vi "v5.vi"() -> ()   [LabVIEW 2022 SP3]
uses:
  <vilib>/DAQmx/read.llb/DAQmx Read (Analog 1D DBL NChan 1Samp).vi
  <vilib>/DAQmx/write.llb/DAQmx Write (Digital Bool 1Line 1Point).vi
  <vilib>/DAQmx/create/channels.llb/DAQmx Create Channel (AI-Voltage-Basic).vi
  <vilib>/DAQmx/create/channels.llb/DAQmx Create Channel (DO-Digital Output).vi
  <vilib>/DAQmx/miscellaneous.llb/DAQmx Fill In Error Info.vi
panel:
  out "Gas detected":bool
  out "flame detected":bool
  in  "lines":tag
  in  "VISA resource name 5":refnum<visa-resource-name>
  out "Fire detected (from camera)":bool
  out "number":i32
  out "data out":string
  in  "Play":bool
  out "Video":picture
  out "error out":errorcluster
  in  "Gas Sensor threshold":dbl
  in  "Temperature Threshold":dbl
  in  "IR sensor threshhold":dbl
  out "temperature voltage output":dbl
  out "MQ2 gas sensor":dbl(knob) scale=0.0..4.0
  out "IR sensor":dbl(knob) scale=2.0..4.0
  out "Temperature":dbl(knob) scale=10.0..60.0
  out "Gas sensor voltage output":dbl
  out "IR sensor voltage output":dbl
  out "Temperatue":dbl
  in  "VISA resource name 4":refnum<visa-resource-name>
  in  "VISA resource name 3":refnum<visa-resource-name>
  in  "VISA resource name":refnum<visa-resource-name>
  in  "VISA resource name 2":refnum<visa-resource-name>
  in  "stop":bool
  in  "physical channels":tag
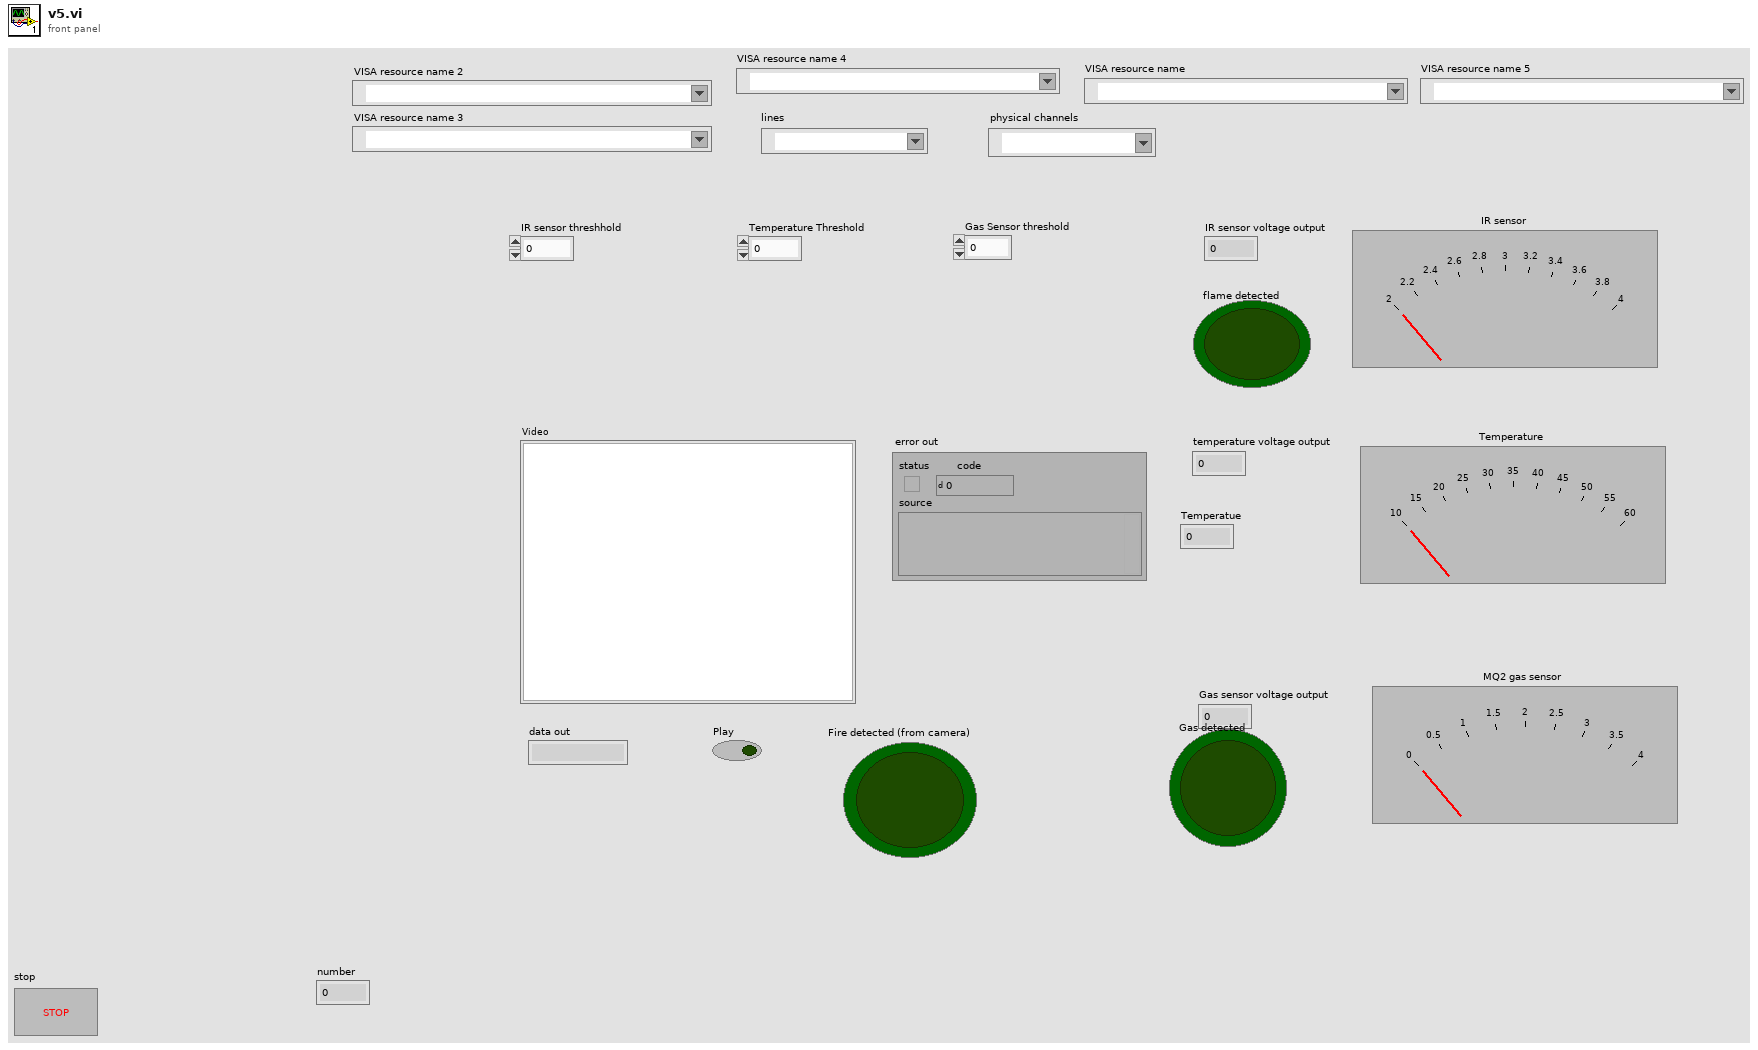
[diagram p1: front panel]
types:
  T1 = enum16{"open", "replace", "create", "open or create", "replace or create", "replace or create with confirmation"}
  T2 = typedef "imagedata.ctl" = cluster{"image type":i32, "image depth":i32, "image":u8[], "mask":u8[], "colors":u32[], "Rectangle":cluster{"left":i16, "top":i16, "right":i16, "bottom":i16}}
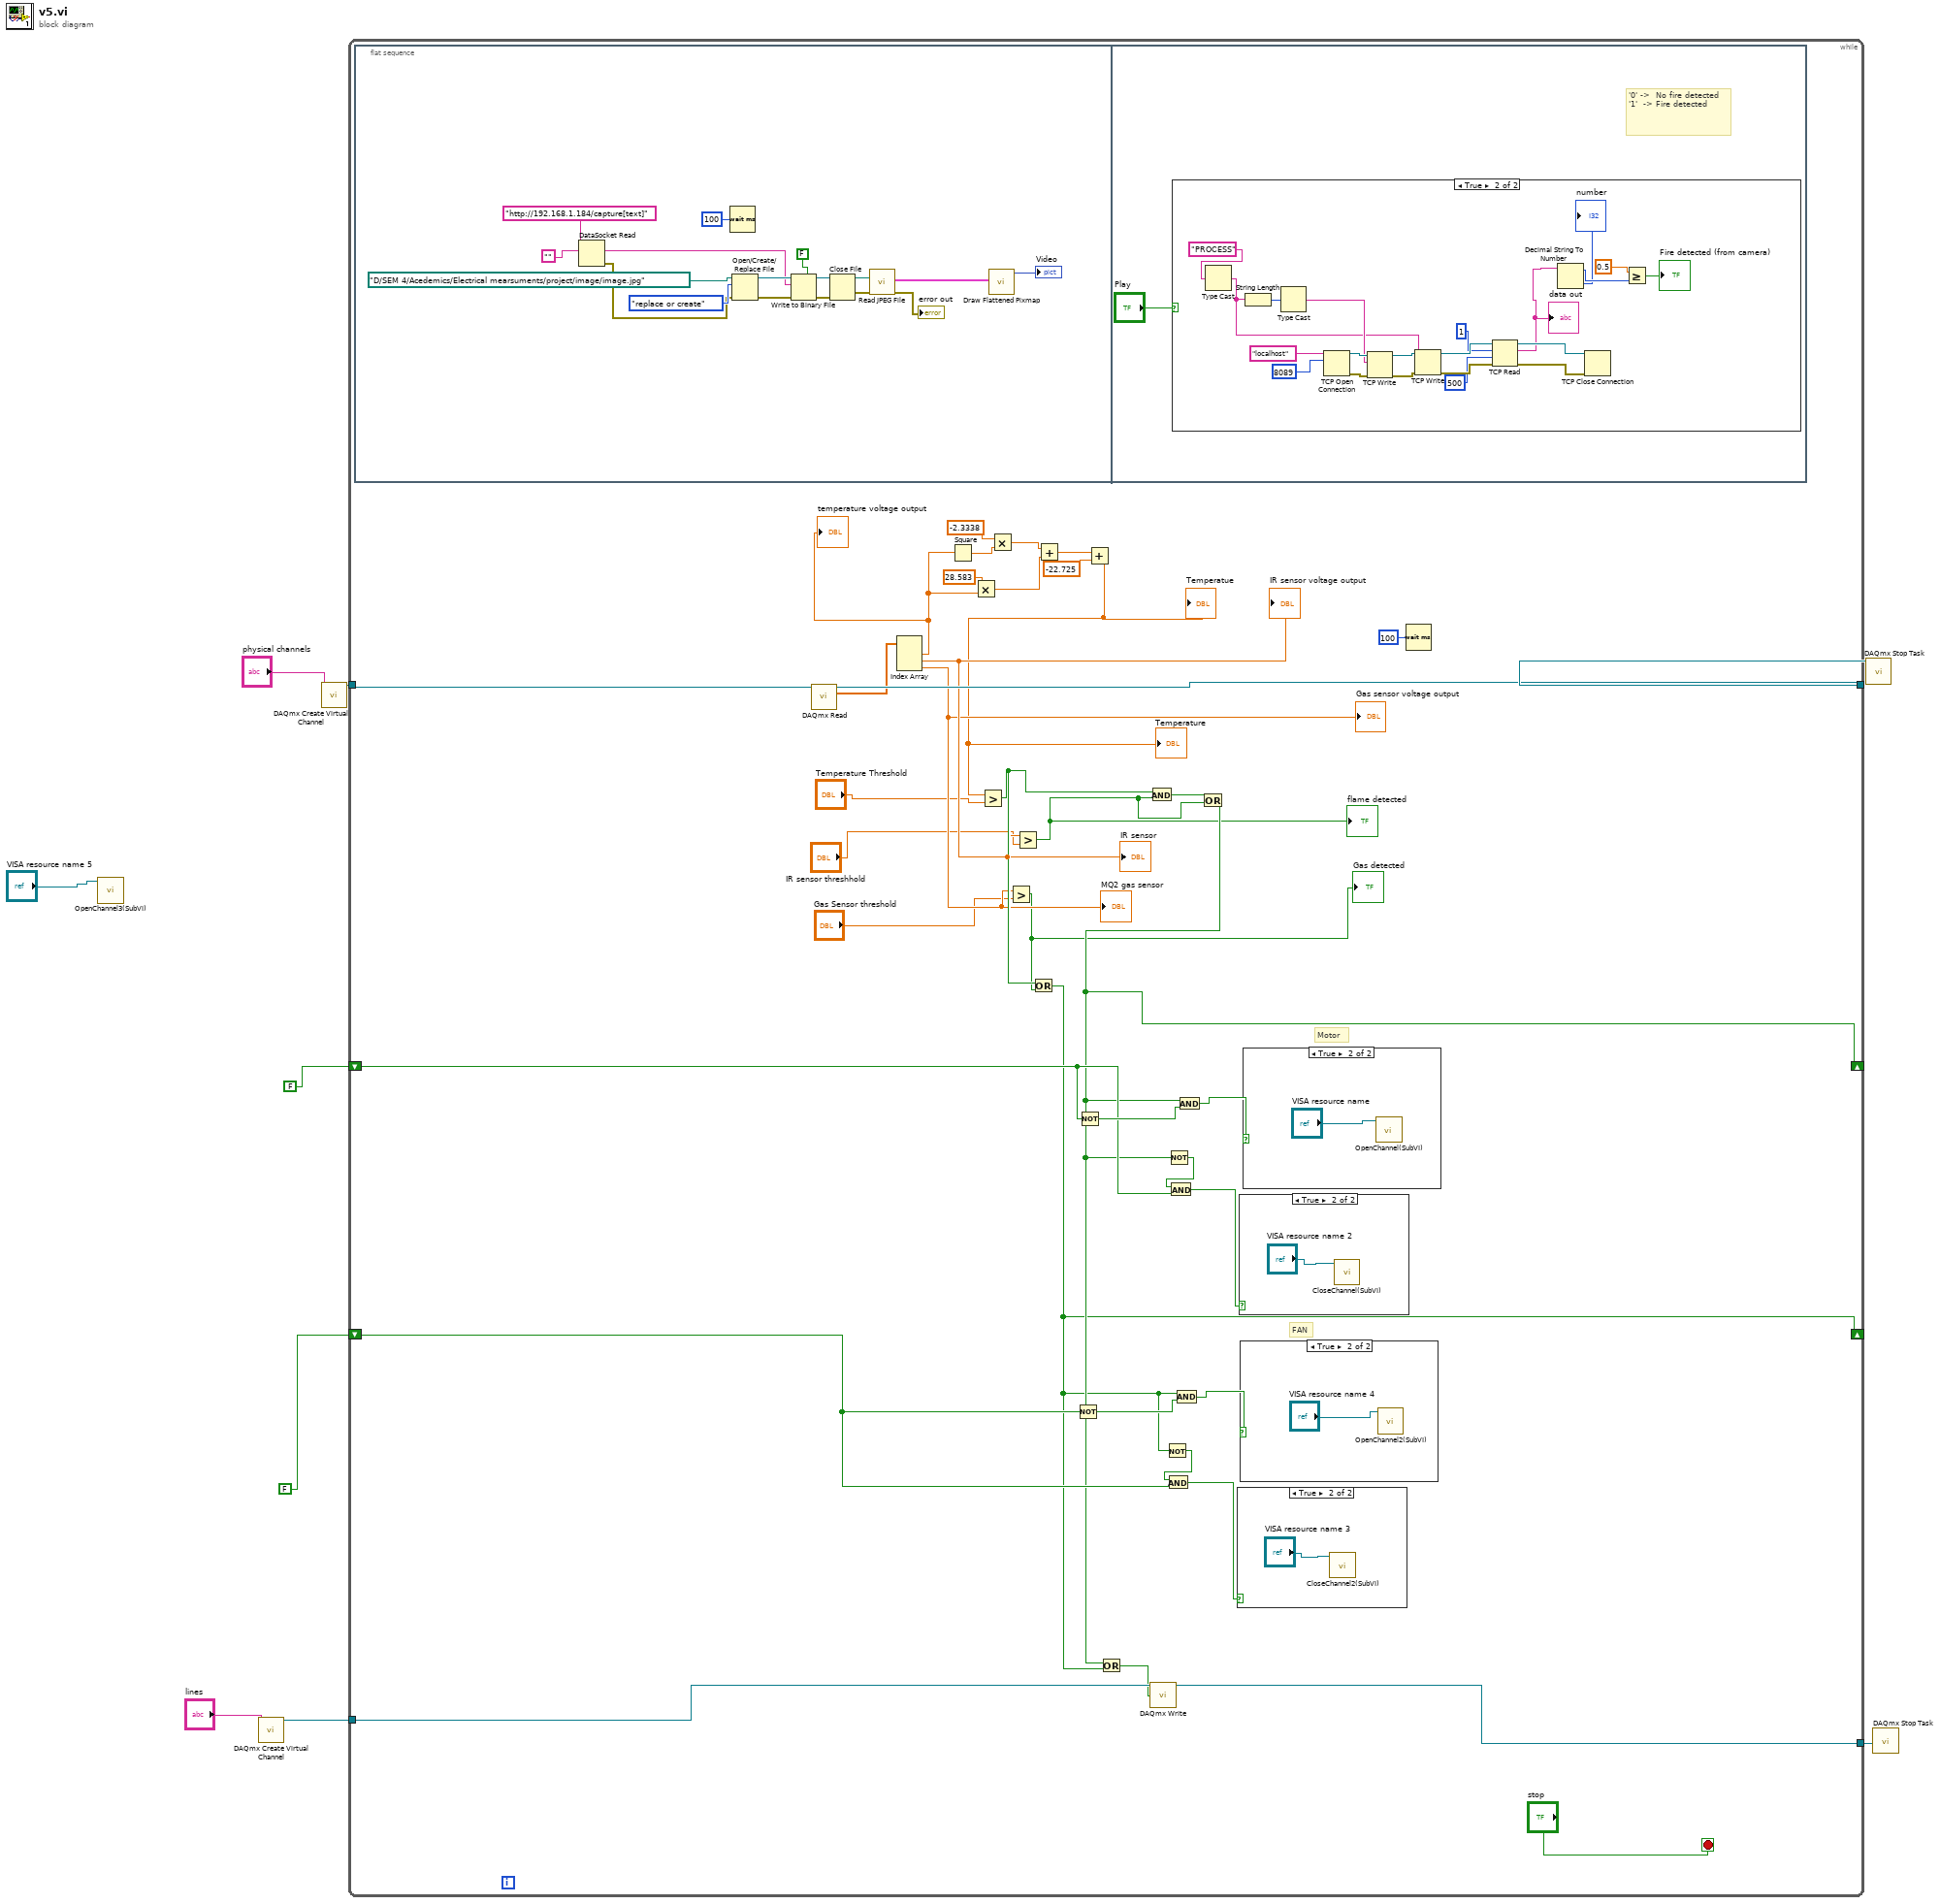
[diagram p0: block diagram]
diagram:
  n1 = call "OpenChannel3(SubVI).vi"("VISA Refnum in"="VISA resource name 5") -> ()  [unwired: 11 in]
  n2 = call-poly <vilib>:"DAQmx Create Virtual Channel.vi"("lines"="lines") -> ("task out"=w2:refnum<k21>)  [unwired: 13 in, 1 out]
  n3 = call-poly <vilib>:"DAQmx Create Virtual Channel.vi"("physical channels"="physical channels") -> ("task out"=w8:refnum<k21>)  [unwired: 13 in, 1 out]
  n4 = while {
    tunnel: w8 -> [w46]
    tunnel: [w45] -> w7
    shift-right: [w16] -> _
    shift-left: FALSE -> [w35]
    shift-right: [w15] -> _
    shift-left: FALSE -> [w34]
    tunnel: w2 -> [w14]
    tunnel: [w13] -> w1
    stop <- "stop" stop-if-true
    # "FAN"
    # "Motor"
    n5 = flat-sequence {
      frame #0 {
        n6 = DataSocket Read(10:"", 11:"http://192.168.1.184/capture[text]") -> (0:w52:errorcluster, 2:w54:string)  [unwired: 1 in, 7 out]
        n7 = Wait (ms)(milliseconds to wait=u32 100) -> ()  [unwired: 1 out]
        n8 = Open/Create/Replace File(file path (use dialog)=path "D:/SEM 4/Acedemics/Electrical mearsuments/project/image/image.jpg", error in=w52, operation (0:open)=T1."replace or create") -> (refnum out=w60:refnum<file>, error out=w61:errorcluster)  [unwired: 3 in, 1 out]
        n9 = Write to Binary File(file (use dialog)=w60, data=w54, error in=w61, 5:FALSE ("prepend array or string size? (T)")) -> (refnum out=w64:refnum<file>, error out=w63:errorcluster)  [unwired: 3 out]
        n10 = Close File(refnum=w64, error in=w63) -> (path=w56:path, error out=w58:errorcluster)
        n11 = call <vilib>:"Read JPEG File.vi"("error in (no error)"=w58, "path to JPEG file"=w56) -> ("error out"=→"error out":errorcluster, "image data"=w51:T2)  [unwired: 8 out]
        n12 = call <vilib>:"Draw Flattened Pixmap.vi"("image data"=w51) -> ("new picture"=→"Video":picture)  [unwired: 1 in, 7 out]
      }
      frame #1 {
        # "'0' ->  No fire detected\n'1'  -> Fire detected"
        n13 = case shown="True" "Play" {
          frame False {
          }
          frame True {
            n14 = Type Cast(x="PROCESS" ("data in")) -> (*(type *) &x=w74:string)  [unwired: 1 out]
            n15 = String Length(string=w74) -> (length=w80:i32)
            n16 = Type Cast(x=w80) -> (*(type *) &x=w75:string)  [unwired: 1 out]
            n17 = TCP Open Connection(address="localhost", remote port or service name=u16 8089) -> (connection ID=w84:refnum<k5>, error out=w83:errorcluster)  [unwired: 3 in]
            n18 = TCP Write(connection ID=w84, data in=w75, error in (no error)=w83) -> (connection ID out=w79:refnum<k5>, error out=w78:errorcluster)  [unwired: 1 in, 1 out]
            n19 = TCP Write(connection ID=w79, data in=w74, error in (no error)=w78) -> (connection ID out=w77:refnum<k5>, error out=w76:errorcluster)  [unwired: 1 in, 1 out]
            n20 = TCP Read(connection ID=w77, bytes to read=1, error in (no error)=w76, 9:500 ("timeout ms (25000)")) -> (connection ID out=w82:refnum<k5>, data out=w71:string, error out=w81:errorcluster)  [unwired: 1 in]
            "data out" <- w71
            n21 = Decimal String To Number(string=w71) -> (offset past number=w68:i32, number=→"number":i32)  [unwired: 2 in]
            n22 = TCP Close Connection(connection ID=w82, error in (no error)=w81) -> ()  [unwired: 1 in, 2 out]
            n23 = Greater Or Equal?(x=0.5, y=w68) -> (x >= y?=→"Fire detected (from camera)":bool)
          }
        }
      }
    }
    n24 = call-poly <vilib>:"DAQmx Read.vi"("task/channels in"=w46) -> ("task out"=w45:refnum<k21>, "data"=w44:dbl[])  [unwired: 12 in, 1 out]
    n25 = Index Array(array=w44) -> (element #1=w21:dbl, element #2=w30:dbl, element #3=w29:dbl)  [unwired: 3 in]
    "IR sensor voltage output" <- w30
    "Gas sensor voltage output" <- w29
    "IR sensor" <- w30
    "MQ2 gas sensor" <- w29
    "temperature voltage output" <- w21
    n26 = Square(x=w21) -> (x^2=w22:dbl)
    n27 = Multiply(x=28.583, y=w21) -> (x*y=w27:dbl)
    n28 = Multiply(x=-2.3338, y=w22) -> (x*y=w26:dbl)
    n29 = Greater?(x=w29, y="Gas Sensor threshold") -> (0:w10:bool)
    "Gas detected" <- w10
    n30 = Greater?(x=w30, y="IR sensor threshhold") -> (0:w11:bool)
    "flame detected" <- w11
    n31 = Add(x=w26, y=w27) -> (x+y=w25:dbl)
    n32 = Not(x=w34) -> (.not. x?=w38:bool)
    n33 = Not(x=w35) -> (.not. x?=w42:bool)
    n34 = Add(x=w25, y=-22.725) -> (x+y=w20:dbl)
    "Temperatue" <- w20
    "Temperature" <- w20
    n35 = Greater?(x=w20, y="Temperature Threshold") -> (0:w32:bool)
    n36 = Or(x=w32, y=w10) -> (x .or. y?=w15:bool)
    n37 = And(x=w32, y=w11) -> (x .and. y?=w31:bool)
    n38 = Not(x=w15) -> (.not. x?=w37:bool)
    n39 = And(x=w37, y=w34) -> (x .and. y?=w36:bool)
    n40 = And(x=w15, y=w38) -> (x .and. y?=w39:bool)
    n41 = Or(x=w11, y=w31) -> (x .or. y?=w16:bool)
    n42 = Or(x=w16, y=w15) -> (x .or. y?=w12:bool)
    n43 = call-poly <vilib>:"DAQmx Write.vi"("task/channels in"=w14, "data"=w12) -> ("task out"=w13:refnum<k21>)  [unwired: 11 in, 2 out]
    n44 = Not(x=w16) -> (.not. x?=w41:bool)
    n45 = And(x=w41, y=w35) -> (x .and. y?=w40:bool)
    n46 = And(x=w16, y=w42) -> (x .and. y?=w43:bool)
    n47 = case shown="True" w36 {
      frame False {
      }
      frame True {
        n48 = call "CloseChannel2(SubVI).vi"("VISA Refnum in"="VISA resource name 3") -> ()  [unwired: 11 in]
      }
    }
    n49 = case shown="True" w40 {
      frame False {
      }
      frame True {
        n50 = call "CloseChannel(SubVI).vi"("VISA Refnum in"="VISA resource name 2") -> ()  [unwired: 11 in]
      }
    }
    n51 = case shown="True" w39 {
      frame False {
      }
      frame True {
        n52 = call "OpenChannel2(SubVI).vi"("VISA Refnum in"="VISA resource name 4") -> ()  [unwired: 11 in]
      }
    }
    n53 = case shown="True" w43 {
      frame False {
      }
      frame True {
        n54 = call "OpenChannel(SubVI).vi"("VISA Refnum in"="VISA resource name") -> ()  [unwired: 11 in]
      }
    }
    n55 = Wait (ms)(milliseconds to wait=u32 100) -> ()  [unwired: 1 out]
  }
  n56 = call <vilib>:"DAQmx Stop Task.vi"("task/channels in"=w7) -> ()  [unwired: 13 in, 2 out]
  n57 = call <vilib>:"DAQmx Stop Task.vi"("task/channels in"=w1) -> ()  [unwired: 13 in, 2 out]
